vi "toggle_pairing_button.vi"(8 "error in":errorcluster, 9 "Setup ID":i32, 10 "settings in":T2[](array[typedef]) {"stim ramp" min=1}, 11 "control cluster in":T1) -> (0 "error out":errorcluster, 3 "settings out":T2[](array[typedef]) {"stim ramp" min=1})   [LabVIEW 2016]
uses:
  Type Definitions/vars_settings.ctl
  Type Definitions/stim_type.ctl
  Type Definitions/backlight_type.ctl
  Type Definitions/control_references.ctl
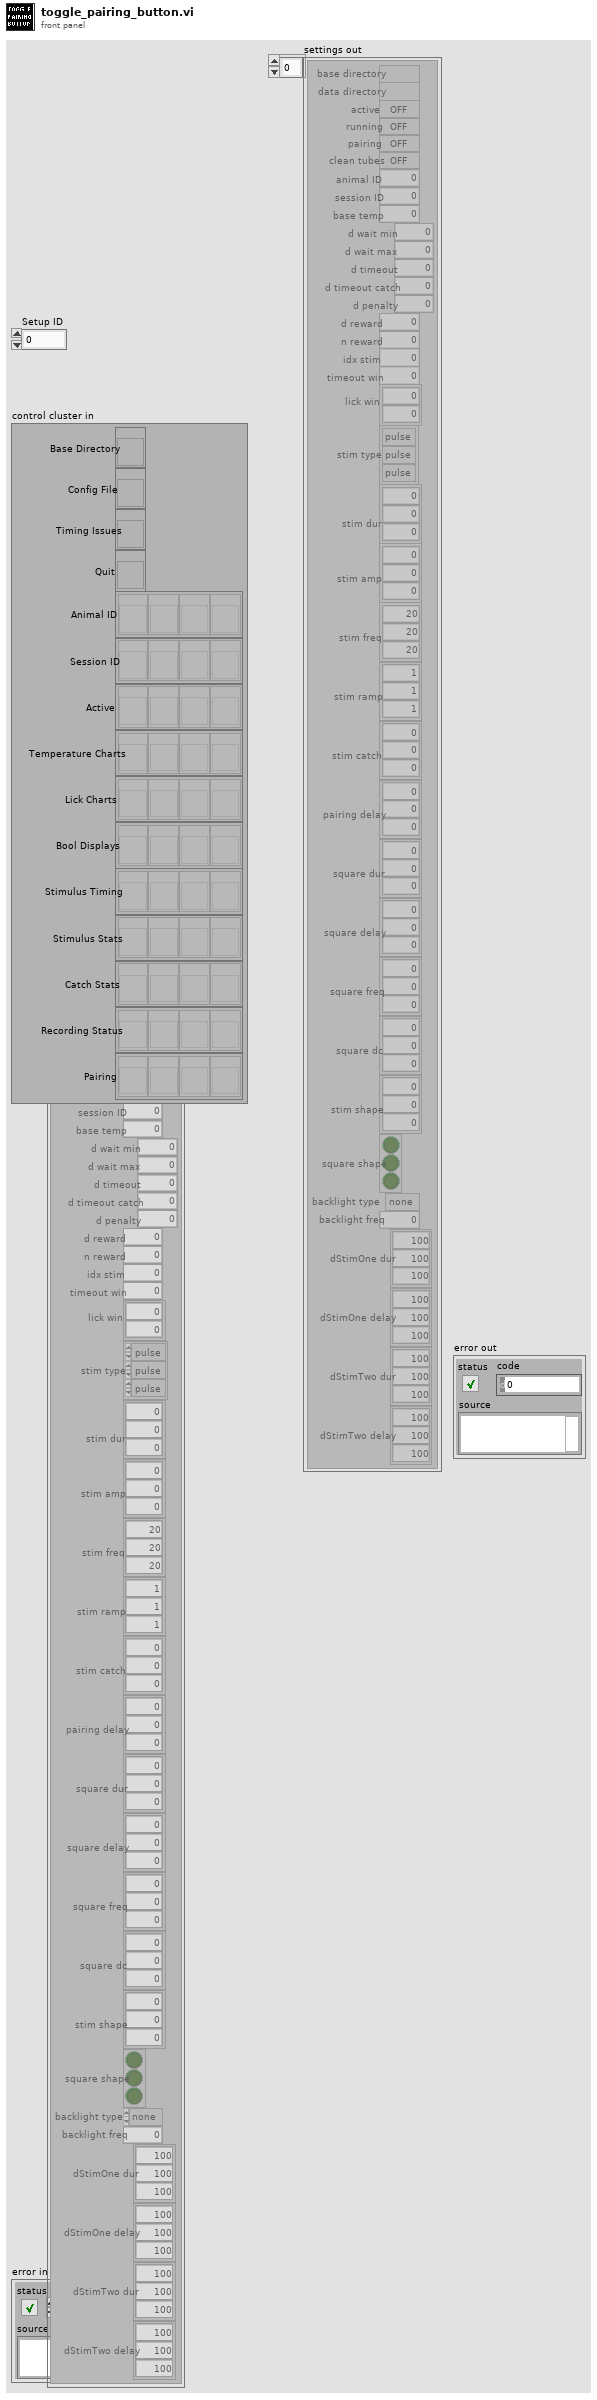
[diagram p1: front panel]
types:
  T1 = typedef "control_references.ctl" = cluster{"Base Directory":refnum<vi>, "Config File":refnum<vi>, "Timing Issues":refnum<vi>, "Quit":refnum<vi>, "Animal ID":refnum<vi>[], "Session ID":refnum<vi>[], "Active":refnum<vi>[], "Temperature Charts":refnum<vi>[], "Lick Charts":refnum<vi>[], "Bool Displays":refnum<vi>[], "Stimulus Timing":refnum<vi>[], "Stimulus Stats":refnum<vi>[], "Catch Stats":refnum<vi>[], "Recording Status":refnum<vi>[], "Pairing":refnum<vi>[]}
  T2 = typedef "vars_settings.ctl" = cluster{"base directory":path, "data directory":path, "active":bool, "running":bool, "pairing":bool, "clean tubes":bool, "animal ID":u16, "session ID":u16, "base temp":dbl, "d wait min":u16, "d wait max":u16, "d timeout":u16, "d timeout catch":u16, "d penalty":u16, "d reward":u16, "n reward":u16, "idx stim":u16, "timeout win":u16, "lick win":i32[], "stim type":T3[], "stim dur":u16[], "stim amp":dbl[], "stim freq":u16[], "stim ramp":u16[], "stim catch":u8[], "pairing delay":i16[], "square dur":u16[], "square delay":i16[], "square freq":u8[], "square dc":u8[], "stim shape":dbl[][], "square shape":bool[][], "backlight type":T4, "backlight freq":u16, "dStimOne dur":u16[], "dStimOne delay":i16[], "dStimTwo dur":u16[], "dStimTwo delay":i16[]}
  T3 = typedef "stim_type.ctl" = enum16{"pulse", "vibration", "square", "sine"}
  T4 = typedef "backlight_type.ctl" = enum16{"none", "random", "regular"}
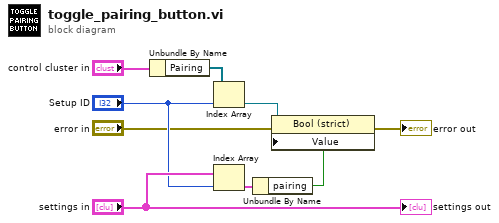
[diagram p0: block diagram]
diagram:
  n1 = Unbundle By Name("control cluster in") -> ("Pairing"=w8:refnum<vi>[])
  n2 = Index Array(array=w8, index="Setup ID") -> (element=w7:refnum<vi>)
  n3 = Index Array(array="settings in", index="Setup ID") -> (element=w9:T2)
  n4 = Unbundle By Name(w9) -> ("pairing"=w3:bool)
  n5 = property class="Bool (strict)"(reference=w7, error in="error in", "Value"=w3) -> (error out=→"error out":errorcluster)  [unwired: 1 out]
  "settings out" <- "settings in"
